vi "Write State.vi"(8 "error in (no error)":errorcluster, 10 "State":string, 11 "Filter_Wheel in":refnum<class "Filter_Wheel.lvclass">) -> (0 "error out":errorcluster, 3 "Filter_Wheel out":refnum<class "Filter_Wheel.lvclass">)   [LabVIEW 2018, in "Filter_Wheel.lvclass"]
uses:
  Filter_Wheel.lvclass
  Filter_Wheel.lvclass/Filter_Wheel.ctl
  State Machine/State Machine.lvclass
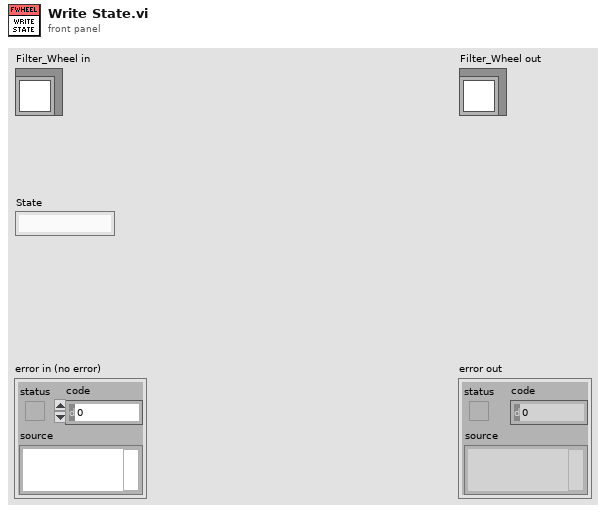
[diagram p1: front panel]
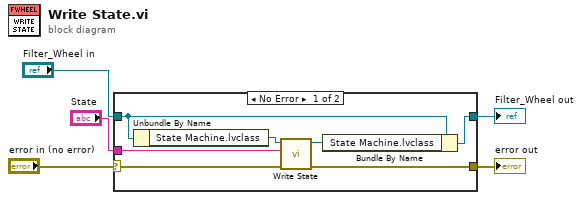
[diagram p0: block diagram]
diagram:
  n1 = case shown="No Error" "error in (no error)" {
    selector: "error in (no error)" -> [w9 w14]
    tunnel: [w8 w14] -> w4
    tunnel: [w11 w13] -> w2
    tunnel: "Filter_Wheel in" -> [w12 w13]
    tunnel: "State" -> [w6 _]
    frame No Error {
      n2 = Unbundle By Name(w12) -> ("State Machine.lvclass"=w10:refnum<class "State Machine.lvclass">)
      n3 = call-dynamic "Write State.vi"("error in (no error)"=w9, "State"=w6, "State Machine in"=w10) -> ("error out"=w8:errorcluster, "State Machine out"=w7:refnum<class "State Machine.lvclass">)  [unwired: 7 in]
      n4 = Bundle By Name(cluster=w12, "State Machine.lvclass"=w7) -> (w11:refnum<class "Filter_Wheel.lvclass">)
    }
    frame Error {
    }
  }
  "error out" <- w4
  "Filter_Wheel out" <- w2
